vi "close serial.vi"(8 "error in (no error)":errorcluster, 11 "SIM_Roda_Filtros in":refnum<class "SIM_Roda_Filtros.lvclass">) -> (0 "error out":errorcluster, 3 "SIM_Roda_Filtros out":refnum<class "SIM_Roda_Filtros.lvclass">)   [LabVIEW 2018, in "SIM_Roda_Filtros.lvclass"]
uses:
  SIM_Roda_Filtros.lvclass
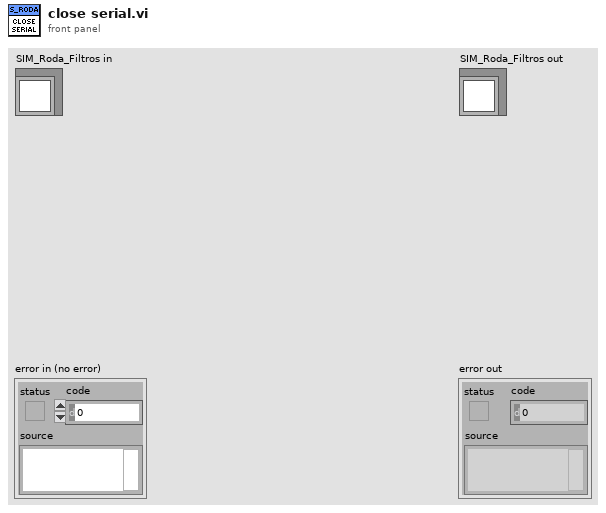
[diagram p1: front panel]
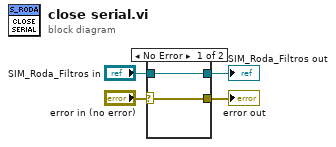
[diagram p0: block diagram]
diagram:
  n1 = case shown="No Error" "error in (no error)" {
    selector: "error in (no error)" -> [w6 w7]
    tunnel: [w6 w7] -> w3
    tunnel: "SIM_Roda_Filtros in" -> [w5 w8]
    tunnel: [w5 w8] -> w1
    frame No Error {
    }
    frame Error {
    }
  }
  "error out" <- w3
  "SIM_Roda_Filtros out" <- w1
